vi "Rescale hist cluster element.vi"(7 "Hist cluster element":i32, 8 "error in (no error)":errorcluster, 9 "Secondary":i32=-1, 10 "Primary":i32=-1, 11 "Hist cluster":T1) -> (0 "error out":errorcluster, 3 "Hist cluster":T1)   [LabVIEW 2016]
uses:
  Typedefs/Coincidence histogram cluster refnum.ctl
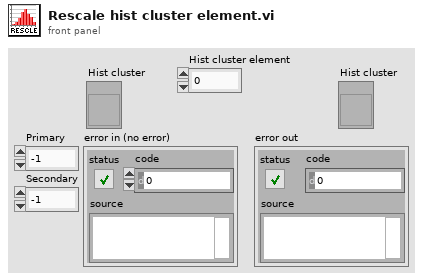
[diagram p1: front panel]
types:
  T1 = typedef "Coincidence histogram cluster refnum.ctl" = refnum<vi>
  T2 = cluster{"X Values":dbl[], "Histogram: h(x)":i32[]}[]
  T3 = cluster{"X Values":dbl[], "Histogram: h(x)":i32[]}
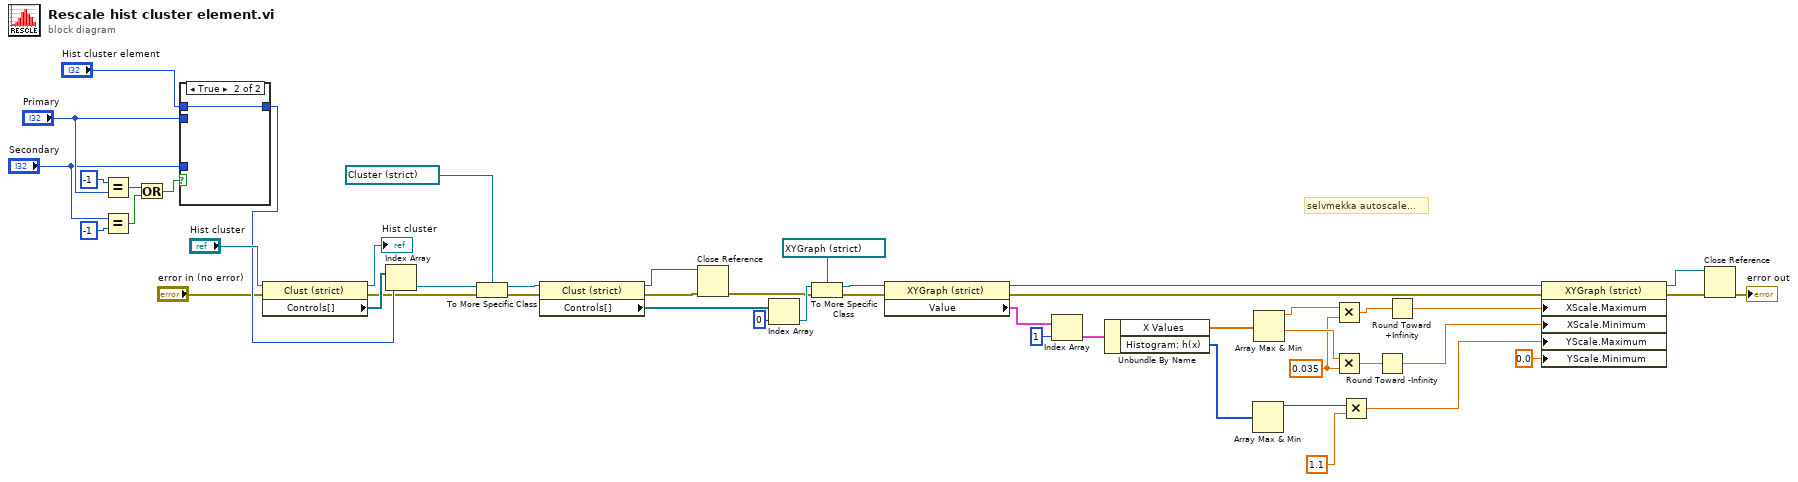
[diagram p0: block diagram]
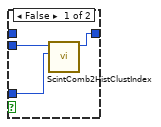
[diagram p2: hidden frame]
diagram:
  w10 = 0.035 ("y")
  # "selvmekka autoscale..."
  n1 = Equal?(x=-1, y="Primary") -> (x = y?=w27:bool)
  n2 = Equal?(x="Secondary", y=-1 ("x")) -> (x = y?=w28:bool)
  n3 = Or(x=w27, y=w28) -> (x .or. y?=w29:bool)
  n4 = case shown="True" w29 {
    tunnel: [w51 w52] -> w41
    tunnel: "Primary" -> [w50 _]
    tunnel: "Secondary" -> [w49 _]
    tunnel: "Hist cluster element" -> [_ w52]
    frame False {
      n5 = call "ScintComb2HistClustIndex.vi"("Secondary"=w49, "Primary"=w50) -> ("Numeric"=w51:i32)  [unwired: 9 in]
    }
    frame True {
    }
  }
  n6 = property class="Clust (strict)"(reference="Hist cluster", error in="error in (no error)") -> (reference out=→"Hist cluster":T1, error out=w40:errorcluster, "Controls[]"=w48:refnum<vi>[])
  n7 = Index Array(array=w48, index=w41) -> (element=w47:refnum<vi>)
  n8 = To More Specific Class(target class=refnum<vi> refnum ("Cluster 2"), reference=w47, error in=w40) -> (specific class reference=w46:refnum<vi>, error out=w39:errorcluster)
  n9 = property on="Property Node" class="Clust (strict)"(reference=w46, error in=w39) -> (reference out=w19:refnum<vi>, error out=w18:errorcluster, "Controls[]"=w45:refnum<vi>[])
  n10 = Close Reference(reference=w19, error in (no error)=w18) -> (error out=w17:errorcluster)
  n11 = Index Array(array=w45, index=0) -> (element=w43:refnum<vi>)
  n12 = To More Specific Class(target class=refnum<vi> refnum ("Histogram Graph"), reference=w43, error in=w17) -> (specific class reference=w23:refnum<vi>, error out=w22:errorcluster)
  n13 = property on="Property Node" class="XYGraph (strict)"(reference=w23, error in=w22) -> (reference out=w20:refnum<vi>, error out=w21:errorcluster, "Value"=w16:T2)
  n14 = Index Array(array=w16, index=1) -> (element=w14:T3)
  n15 = Unbundle By Name(w14) -> ("X Values"=w13:dbl[], "Histogram: h(x)"=w5:i32[])
  n16 = Array Max & Min(array=w5) -> (max value=w4:i32)  [unwired: 3 out]
  n17 = Array Max & Min(array=w13) -> (max value=w12:dbl, min value=w11:dbl)  [unwired: 2 out]
  n18 = Multiply(x=w12, y=w10) -> (x*y=w9:dbl)
  n19 = Multiply(x=w11, y=w10) -> (x*y=w7:dbl)
  n20 = Multiply(x=w4, y=1.1) -> (x*y=w2:dbl)
  n21 = Round Toward -Infinity(1:w7) -> (0:w6:dbl)
  n22 = Round Toward +Infinity(x=w9) -> (ceil(x): smallest int >= x=w8:dbl)
  n23 = property on="Property Node" class="XYGraph (strict)"(reference=w20, error in=w21, "XScale.Maximum"=w8, "XScale.Minimum"=w6, "YScale.Maximum"=w2, "YScale.Minimum"=0.0 ("Y Scale.Range:Minimum")) -> (reference out=w36:refnum<vi>, error out=w35:errorcluster)
  n24 = Close Reference(reference=w36, error in (no error)=w35) -> (error out=→"error out":errorcluster)
